vi "Set Jog Low Speed.vi"(4 "error in (no error)":errorcluster, 5 "Jog Low Speed (0 units/s)":dbl min=0.0 format="%.6f", 6 "Axis (1)":i32=1 min=1 max=3, 7 "VISA resource name":refnum<visa-resource-name>) -> (0 "error out":errorcluster, 3 "VISA resource name out":refnum<visa-resource-name>)   [LabVIEW 2020, in "Newport ESP301.lvlib"]
doc: "This command is used to set the low speed for jogging an axis. Its execution is immediate, meaning that the value is changed when the command is processed, including when motion is in progress. It can be used as an immediate command or inside a program."
uses:
  Newport ESP301.lvlib
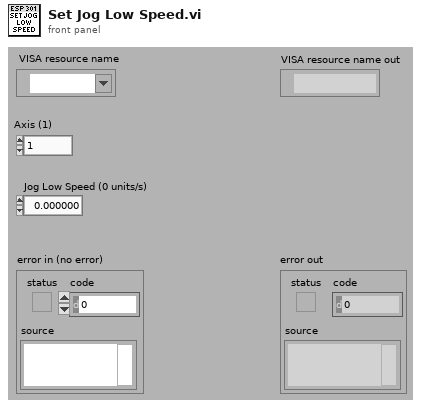
[diagram p1: front panel]
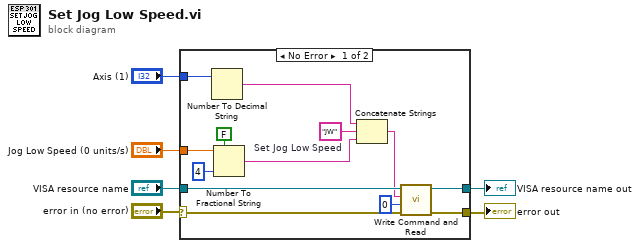
[diagram p0: block diagram]
diagram:
  n1 = case shown="No Error" "error in (no error)" {
    selector: "error in (no error)" -> [w16 w21]
    tunnel: [w18 w21] -> w6
    tunnel: "VISA resource name" -> [w19 w20]
    tunnel: [w17 w20] -> w5
    tunnel: "Axis (1)" -> [w11 _]
    tunnel: "Jog Low Speed (0 units/s)" -> [w10 _]
    frame No Error {
      w15 = "JW"  # Set Jog Low Speed
      n2 = Number To Decimal String(number=w11) -> (decimal integer string=w12:string)  [unwired: 1 in]
      n3 = Number To Fractional String(use system decimal point (T)=FALSE ("utiliser le séparateur décimal du système (V)"), number=w10, precision (6)=i16 4 ("précision (6)")) -> (F-format string=w14:string)  [unwired: 1 in]
      n4 = Concatenate Strings(w12, w15, w14) -> (w9:string)
      n5 = call "Write Command and Read.vi"("error in (no error)"=w16, "Bytes to read (100)"=u32 0, "Command"=w9, "VISA resource name"=w19) -> ("error out"=w18:errorcluster, "VISA resource name out"=w17:refnum<visa-resource-name>)  [unwired: 3 in, 1 out]
    }
    frame Error {
    }
  }
  "error out" <- w6
  "VISA resource name out" <- w5
